vi "io_refnum.vi"() -> ()   [LabVIEW 2020]
panel:
  in  "sv":refnum<k21>
  in  "visa":refnum<visa-resource-name>
  in  "ivi":refnum<k15>
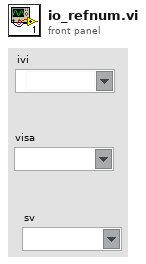
[diagram p1: front panel]
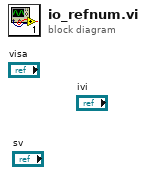
[diagram p0: block diagram]
diagram:
